vi "TagBus_Create Tags from Controls.vi"(10 "Array":refnum<vi>[](array[refnum]), 11 "Process Name":string) -> (3 "TagDescriptions":refnum<class "tag descriptor.lvclass">[](array[class]))   [LabVIEW 2015, in "TagBus.lvclass"]
uses:
  TagBus.lvclass
  <vilib>/NI/Tag Bus/tag/tag descriptor.lvclass
  <vilib>/NI/Tag Bus/tag/Data Type.ctl
  <vilib>/Utility/Data Type/NI_Data Type.lvlib
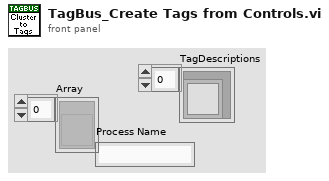
[diagram p1: front panel]
types:
  T1 = typedef "tag bus.lvlib/tag descriptor.lvclass/Data Type.ctl" = enum16{"Double", "Single", "I64", "I32", "I16", "I8", "U64", "U32", "U16", "U8", "Boolean", "String", "Array of Double", "Array of Single", "Array of I64", "Array of I32", "Array of I16", "Array of I8", "Array of U64", "Array of U32", "Array of U16", "Array of U8", "Array of Boolean", "Array of String"}
  T2 = typedef "NI_Data Type.lvlib/Data Type.ctl" = enum8{"Invalid Type", "Void", "I8", "I16", "I32", "I64", "U8", "U16", "U32", "U64", "Single Float", "Double Float", "Extended Float", "Single Complex", "Double Complex", "Extended Complex", "Enum U8", "Enum U16", "Enum U32", "Enum U64", "Single Float With Unit", "Double Float With Unit", "Extended Float With Unit", "Single Complex with Unit", "Double Complex with Unit", "Extended Complex with Unit", "Boolean", "String", "Path", "Picture", "Tag", "Array", "Cluster", "Variant", "LV Variant", "Waveform", "Timestamp", "Digital Waveform", "Digital Data", "ExpressData", "Refnum", "External Data", "VI", "Poly VI", "LabVIEW Class Instance", "Fixed Point"}
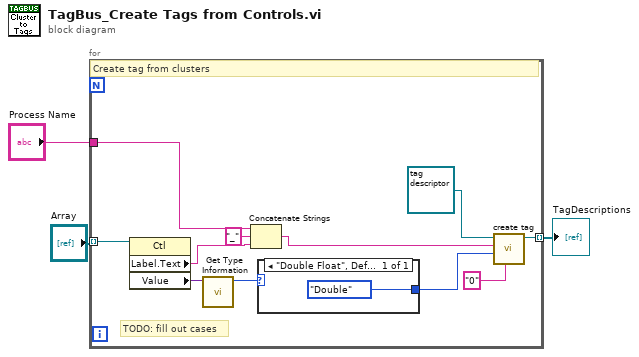
[diagram p0: block diagram]
diagram:
  n1 = for {
    tunnel: "Array" -> [w14] mode=indexing
    tunnel: [w12] -> w2 mode=indexing
    tunnel: "Process Name" -> [w7]
    # "TODO: fill out cases"
    # "Create tag from clusters"
    n2 = property class="Ctl"(reference=w14) -> ("Label.Text"=w9:string, "Value"=w13:variant)  [unwired: 1 in, 2 out]
    n3 = call <vilib>:"Get Type Information.vi"("Variant"=w13) -> ("Type"=w5:T2)  [unwired: 6 in, 4 out]
    n4 = Concatenate Strings(w7, "_" ("string"), w9) -> (w8:string)
    n5 = case shown="\"Double Float\", Default" w5 {
      tunnel: [Data_Type."Double" ("data type")] -> w4
      frame "Double Float", Default {
      }
    }
    n6 = call-dynamic "create tag.vi"("raw default"="0", "data type"=w4, "name"=w8, "tag descriptor in"=refnum<class "tag descriptor.lvclass"> refnum) -> ("tag descriptor out"=w12:refnum<class "tag descriptor.lvclass">)  [unwired: 6 in, 1 out]
  }
  "TagDescriptions" <- w2
